vi "PulseTrain.vi"(8 "error in":errorcluster, 10 "duty cycle":dbl format="%.6f", 11 "frequency":dbl format="%.6f") -> (0 "error out":errorcluster, 3 "task out":refnum<k21>)   [LabVIEW 2009]
uses:
  <vilib>/DAQmx/create/channels.llb/DAQmx Create Channel (CO-Pulse Generation-Frequency).vi
  <vilib>/DAQmx/configure/timing.llb/DAQmx Timing (Implicit).vi
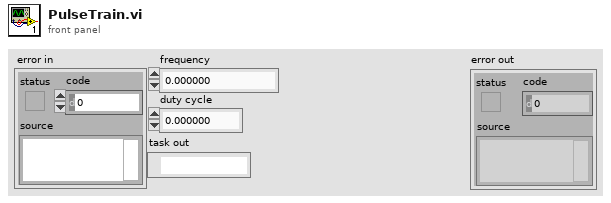
[diagram p1: front panel]
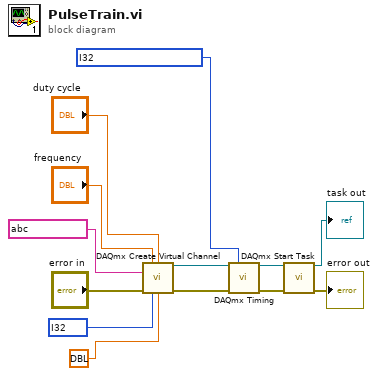
[diagram p0: block diagram]
diagram:
  w1 = i32 ? items=["Finite Samples", "Continuous Samples", "Hardware Timed Single Point"] ("sample mode")
  w9 = i32 ? items=["High", "Low"] ("idle state")
  n1 = call-poly <vilib>:"DAQmx Create Virtual Channel.vi"("frequency"="frequency", "duty cycle"="duty cycle", "counter"=tag ?, "error in"="error in", "idle state"=w9, "initial delay"=dbl ?) -> ("task out"=w5:refnum<k21>, "error out"=w2:errorcluster)  [unwired: 8 in]
  n2 = call-poly <vilib>:"DAQmx Timing.vi"("task/channels in"=w5, "sample mode"=w1, "error in"=w2) -> ("task out"=w4:refnum<k21>, "error out"=w3:errorcluster)  [unwired: 11 in]
  n3 = call <vilib>:"DAQmx Start Task.vi"("task/channels in"=w4, "error in"=w3) -> ("task out"=→"task out":refnum<k21>, "error out"=→"error out":errorcluster)  [unwired: 12 in]
